vi "mean_.vi"   [LabVIEW 2010]
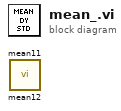
[diagram p0: block diagram]
diagram:
  n1 = call "mean12.vi"() -> ()  [unwired: 6 in, 3 out]
  n2 = call "mean11.vi"() -> ()  [unwired: 6 in, 3 out]
